vi "Valid Self Defined Pattern or Not.vi"(8 "error in (no error)":errorcluster, 10 "self defined pattern":enum16{"5 X 10", "5 X 8"}(ring), 11 "customized character pattern":bool[][](array[boolean])) -> (0 "error out":errorcluster)   [LabVIEW 2017, in "HD44780.lvclass"]
uses:
  HD44780.lvclass
  Common/HD44780 Common.lvlib
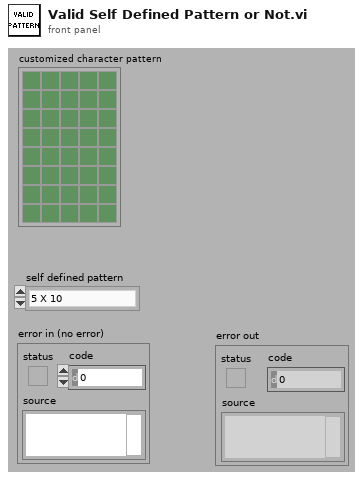
[diagram p1: front panel]
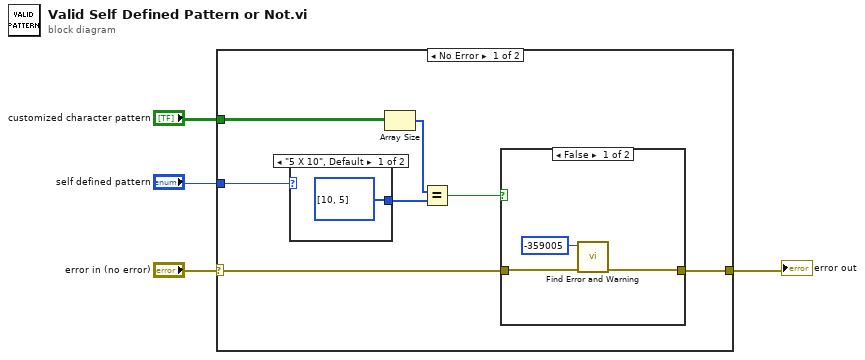
[diagram p0: block diagram]
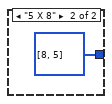
[diagram p3: hidden frame]
diagram:
  n1 = case shown="No Error" "error in (no error)" {
    selector: "error in (no error)" -> [w9 w18]
    tunnel: [w8 w18] -> w3
    tunnel: "customized character pattern" -> [w6 _]
    tunnel: "self defined pattern" -> [w5 _]
    frame No Error {
      n2 = case shown="\"5 X 10\", Default" w5 {
        tunnel: [i32[] [10, 5] ("y") i32[] [8, 5] ("y")] -> w10
        frame "5 X 10", Default {
        }
        frame "5 X 8" {
        }
      }
      n3 = Array Size(array=w6) -> (size(s)=w11:i32[])
      n4 = Equal?(x=w11, y=w10) -> (x = y?=w7:bool)
      n5 = case shown="False" w7 {
        tunnel: w9 -> [w12 w15]
        tunnel: [w13 w15] -> w8
        frame False {
          n6 = call "Find Error and Warning.vi"("error in (no error)"=w12, "error code"=-359005) -> ("error out"=w13:errorcluster)  [unwired: 9 in]
        }
        frame True {
        }
      }
    }
    frame Error {
    }
  }
  "error out" <- w3
